vi "UI Manager_Create.vi"(0 "reference in":refnum<class "UI Manager.lvclass">, 5 "Error In":errorcluster) -> (14 "reference out":refnum<class "UI Manager.lvclass">, 19 "Error Out":errorcluster)   [LabVIEW 2024, in "UI Manager.lvclass"]
uses:
  UI Manager.lvclass
  C:/Users/burakkorkmaz/Desktop/Leveling/labview-desing-patterns/Proxy Pattern/User Manager_class/User Manager.lvclass
  UI Manager.lvclass/UI Manager.ctl
  User Manager_class/User Manager.lvclass
  C:/Users/burakkorkmaz/Desktop/Leveling/labview-desing-patterns/Proxy Pattern/UI Manager_class/UI Manager.lvclass
panel:
  # "Connector Pane"
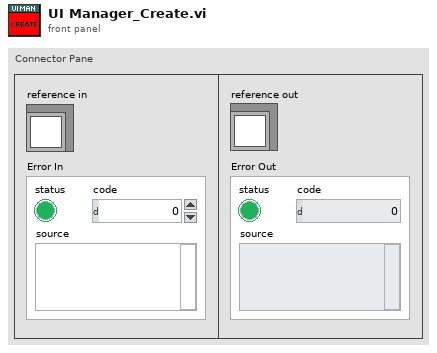
[diagram p1: front panel]
types:
  T1 = typedef "UI Manager.lvclass/ObjectAttributes.ctl" = cluster{"None":bool}
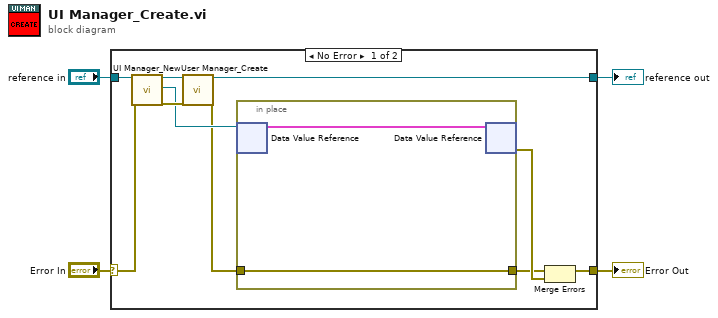
[diagram p0: block diagram]
diagram:
  n1 = case shown="No Error" "Error In" {
    selector: "Error In" -> [w13 w18]
    tunnel: [w11 w18] -> w3
    tunnel: "reference in" -> [w14 w17]
    tunnel: [w8 w17] -> w1
    frame No Error {
      n2 = call "UI Manager_New.vi"("reference in"=w14, "Error In"=w13) -> ("reference out"=w10:refnum<class "UI Manager.lvclass">, "DVRRefOut"=w7:refnum<data-value>, "Error Out"=w9:errorcluster)  [unwired: 14 in, 1 out]
      n3 = call "User Manager_Create.vi"("reference in"=w10, "Error In"=w9) -> ("reference out"=w8:refnum<class "UI Manager.lvclass">, "Error Out"=w6:errorcluster)  [unwired: 16 in]
      n4 = in-place {
        in-place-border: w6 -> [w15]
        in-place-border: [w15] -> w5
        n5 = in-place-dvr #1(w7) -> (w16:T1)  [unwired: 1 out]
        n6 = in-place-dvr #1(w16) -> (w12:errorcluster)  [unwired: 1 out]
      }
      n7 = Merge Errors(w5, w12) -> (w11:errorcluster)
    }
    frame Error {
    }
  }
  "Error Out" <- w3
  "reference out" <- w1
